vi "Set configuration chain.vi"(8 "error in (no error)":errorcluster, 9 "class names":string[](array[string]), 10 "configuration":variant[](array[variant]), 11 "BMC in":refnum<class "BMC.lvclass">) -> (0 "error out":errorcluster, 3 "BMC out":refnum<class "BMC.lvclass">)   [LabVIEW 2012, in "BMC.lvclass"]
uses:
  BMC.lvclass
  <vilib>/Distrio/Murmex/Murmex/Murmex.lvclass
  BMC.lvclass/BMC.ctl
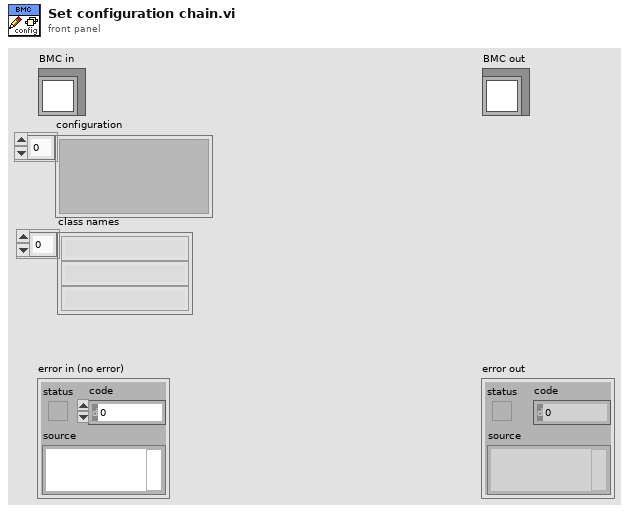
[diagram p1: front panel]
types:
  T1 = typedef "BMC.lvclass/configuration_cluster.ctl" = cluster{"Mapping file":path, "Flat mirror file":path}
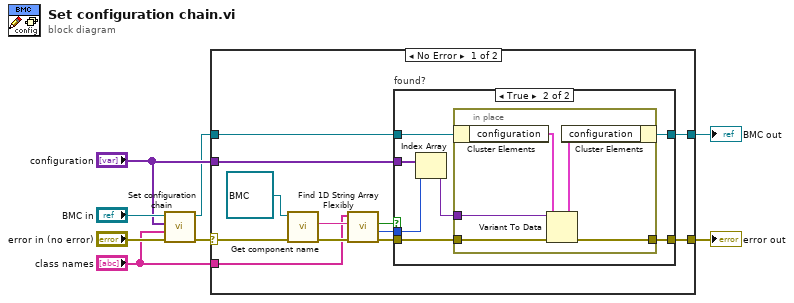
[diagram p0: block diagram]
diagram:
  n1 = call-parent "Set configuration chain.vi"("error in (no error)"="error in (no error)", "class names"="class names", "configuration"="configuration", "Murmex in"="BMC in") -> ("error out"=w6:errorcluster, "Murmex out"=w3:refnum<class "BMC.lvclass">)  [unwired: 6 in]
  n2 = case shown="No Error" w6 {
    selector: w6 -> [w19 w35]
    tunnel: "class names" -> [w16 _]
    tunnel: "configuration" -> [w12 _]
    tunnel: w3 -> [w11 w36]
    tunnel: [w10 w35] -> w2
    tunnel: [w9 w36] -> w1
    frame No Error {
      n3 = call <vilib>:"Get component name.vi"("error in (no error)"=w19, "Murmex in"=refnum<class "BMC.lvclass"> refnum ("BMC")) -> ("error out"=w18:errorcluster, "component name"=w17:string)  [unwired: 7 in, 1 out]
      n4 = call <vilib>:"Find 1D String Array Flexibly.vi"("error in (no error)"=w18, "element"=w17, "array"=w16) -> ("error out"=w15:errorcluster, "index of element"=w13:i32, "found?"=w14:bool)  [unwired: 6 in]
      n5 = case "found?" shown="True" w14 {
        tunnel: w13 -> [_ w27]
        tunnel: w15 -> [w22 w26]
        tunnel: [w22 w25] -> w10
        tunnel: [w21 w23] -> w9
        tunnel: w11 -> [w21 w29]
        tunnel: w12 -> [_ w28]
        frame False {
        }
        frame True {
          n6 = Index Array(array=w28, index=w27) -> (element=w24:variant)
          n7 = in-place {
            in-place-border: w26 -> [w34]
            in-place-border: [w33] -> w25
            in-place-border: w24 -> [w30]
            n8 = in-place-cluster #1(w29) -> ("configuration"=w32:T1)
            n9 = Variant To Data(error in=w34, type=w32, Variant=w30) -> (data=w31:T1, error out=w33:errorcluster)
            n10 = in-place-cluster #1("configuration"=w31) -> (w23:refnum<class "BMC.lvclass">)
          }
        }
      }
    }
    frame Error {
    }
  }
  "error out" <- w2
  "BMC out" <- w1
